vi "MultiStation@SetStationON__Parameter.vi"(1 "ParamterIn":string) -> (0 "ParamterOut":string)   [LabVIEW 2020]
panel:
  in  "IDName":string(combo)
  in  "StationName":string(combo)
  in  "Confirm":bool
  # "MultiStation@SetStationON $Station.$ID"
  # "."
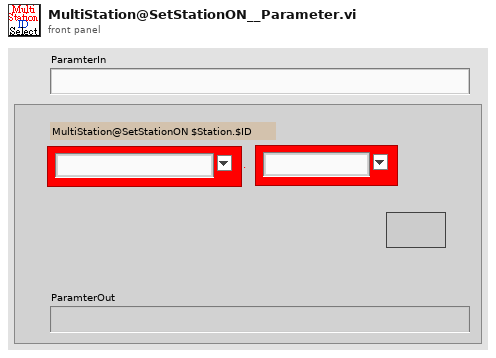
[diagram p1: front panel]
types:
  T1 = enum16{"Init", "AddStation", "StateShift", "ResetDefault", "SetStationON", "SetStationOFF", "SetStationOK", "SetStationNG", "UpdateIndicator", "SetData", "GetData", "GetOnOff", "GetOkNg", "ShowFeedInTray", "ShowFeedOutTray", "BlinkingOn", "BlinkingOff"}
  T2 = cluster{"轉盤燈號":refnum<vi>[], "各站資料":cluster{"轉盤燈號":bool, "錯誤燈號":bool, "資料":variant}[], "IDList":string[]}[]
  T3 = cluster{"轉盤燈號":refnum<vi>[], "各站資料":cluster{"轉盤燈號":bool, "錯誤燈號":bool, "資料":variant}[], "IDList":string[]}
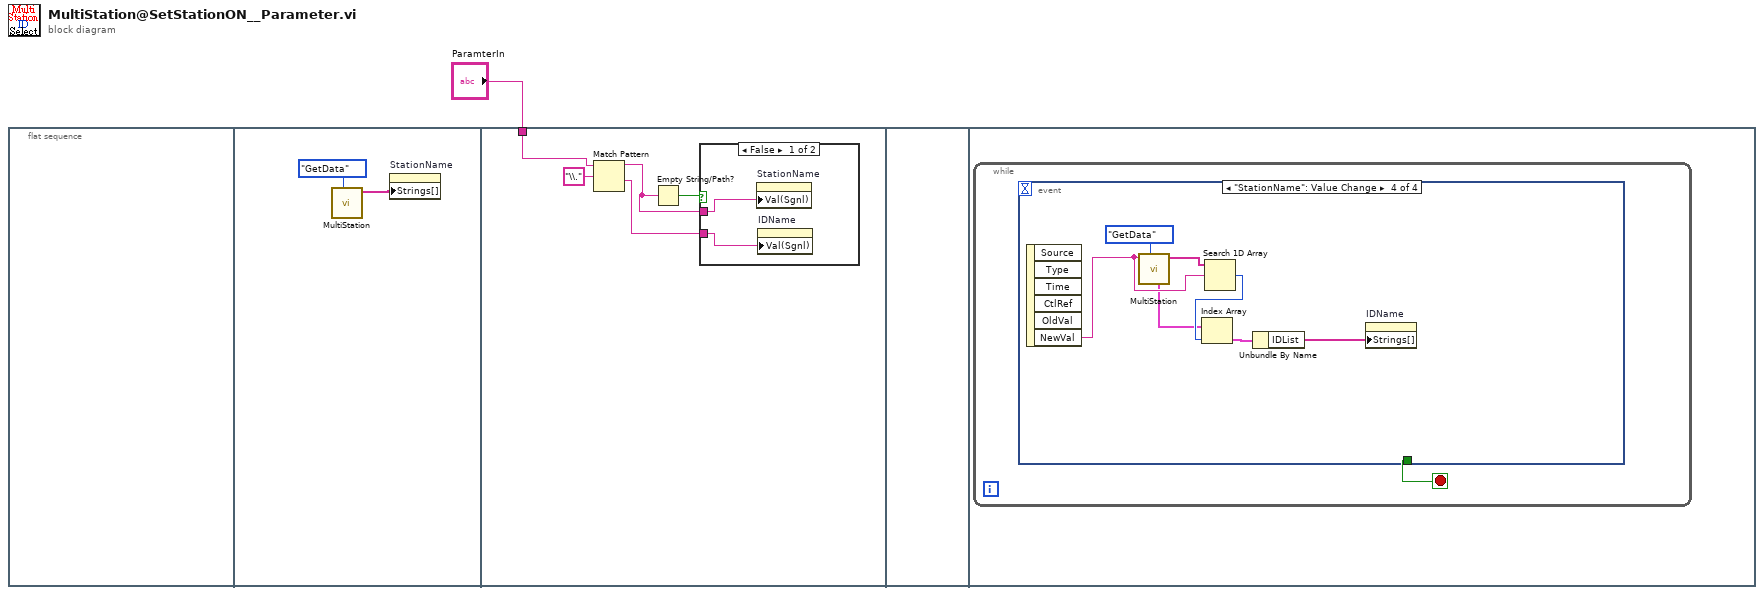
[diagram p0: block diagram]
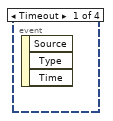
[diagram p3: hidden frame]
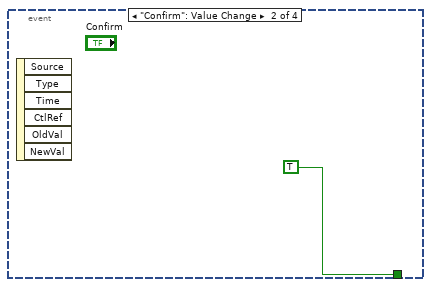
[diagram p4: hidden frame]
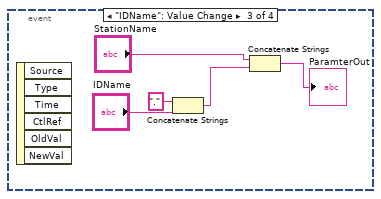
[diagram p5: hidden frame]
diagram:
  n1 = flat-sequence {
    tunnel: "ParamterIn" -> [w4]
    frame #0 {
    }
    frame #1 {
      n2 = call "MultiStation.vi"("OP"=T1."GetData") -> ("StationList"=w2:string[])  [unwired: 6 in, 4 out]
      n3 = property on="StationName" class="CmbBox"("Strings[]"=w2) -> ()  [unwired: 2 in, 2 out]
    }
    frame #2 {
      n4 = Match Pattern(string=w4, regular expression="\\.") -> (before substring=w6:string, after substring=w5:string)  [unwired: 1 in, 2 out]
      n5 = Empty String/Path?(string/path=w6) -> (empty?=w8:bool)
      n6 = case shown="False" w8 {
        tunnel: w6 -> [w10 _]
        tunnel: w5 -> [w9 _]
        frame False {
          n7 = property on="StationName" class="CmbBox"("Val(Sgnl)"=w10) -> ()  [unwired: 2 in, 2 out]
          n8 = property on="IDName" class="CmbBox"("Val(Sgnl)"=w9) -> ()  [unwired: 2 in, 2 out]
        }
        frame True {
        }
      }
    }
    frame #3 {
    }
    frame #4 {
      n9 = while {
        stop <- w11 stop-if-true
        n10 = event shown="[3] \"StationName\": Value Change" {
          selector: _ -> [_ _ _ _]
          dyn-events: _ -> [_ _ _ _]
          timeout: _ -> [_ _ _ _]
          tunnel: [_ TRUE _ _] -> w11
          event Timeout {
            n11 = event-data() -> ()  [unwired: 1 in, 3 out]
          }
          event "Confirm": Value Change {
            n12 = event-data() -> ()  [unwired: 1 in, 6 out]
          }
          event "IDName": Value Change {
            n13 = event-data() -> ()  [unwired: 1 in, 6 out]
            n14 = Concatenate Strings("." ("string"), "IDName") -> (w13:string)
            n15 = Concatenate Strings("StationName", w13) -> (→"ParamterOut":string)
          }
          event "StationName": Value Change {
            n16 = event-data() -> ("NewVal"=w22:string)  [unwired: 1 in, 5 out]
            n17 = call "MultiStation.vi"("OP"=T1."GetData", "StationID"=w22) -> ("StationList"=w23:string[], "StationInfoS"=w20:T2)  [unwired: 5 in, 3 out]
            n18 = Search 1D Array(1D array=w23, element=w22) -> (index of element=w21:i32)  [unwired: 1 in]
            n19 = Index Array(array=w20, index=w21) -> (element=w19:T3)
            n20 = Unbundle By Name(w19) -> ("IDList"=w18:string[])
            n21 = property on="IDName" class="CmbBox"("Strings[]"=w18) -> ()  [unwired: 2 in, 2 out]
          }
        }
      }
    }
  }
